vi "Configure FP-Message-Image.vi"(5 "header ref":refnum<vi>, 7 "Pop Up ref":refnum<vi>, 8 "error in (no error)":errorcluster, 9 "Image ref":refnum<vi>, 10 "Message ref":refnum<vi>, 11 "Popup in":refnum<class "Popup.lvclass">) -> (0 "error out":errorcluster, 2 "Panel Ref":refnum<vi>, 3 "Popup out":refnum<class "Popup.lvclass">, 4 "Panel Width":i32, 6 "Panel Height":i32)   [LabVIEW 2021, in "Pop-Up.lvlib" / "Popup.lvclass"]
doc: "Configure the front panel size, the message, and the image for a custom pop up type.\n\n<b>Code Developed By:</b>\nTechnology Service Corporation\n1983 S Liberty Drive\nBloomington, IN 47403\nPhone: 812 558-7100\nwww.tsc.com/atcs\n\nDeveloper:\nDaniel Coons"
uses:
  Popup.lvclass
  Popup.lvclass/Popup.ctl
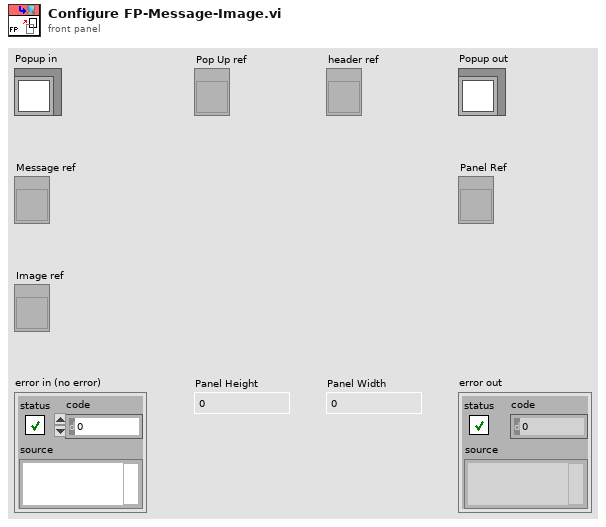
[diagram p1: front panel]
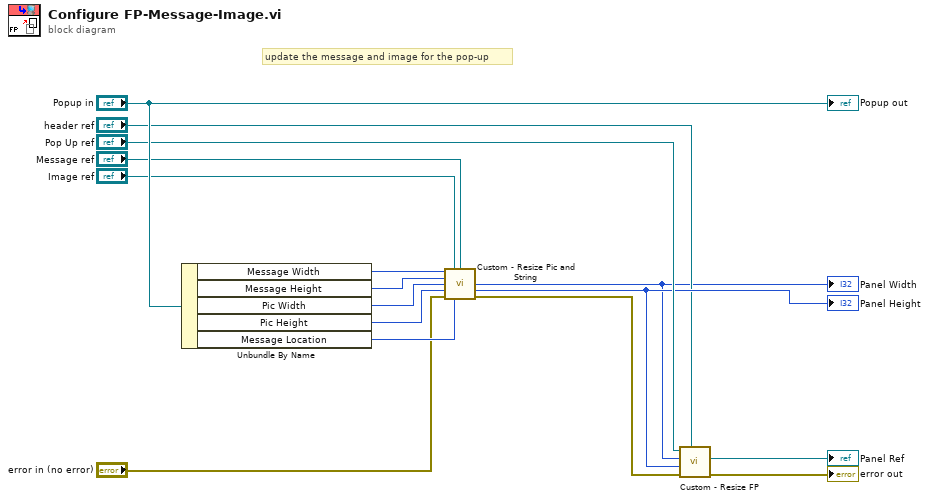
[diagram p0: block diagram]
diagram:
  # "update the message and image for the pop-up"
  n1 = Unbundle By Name("Popup in") -> ("Message Width"=w11:i32, "Message Height"=w12:i32, "Pic Width"=w13:i16, "Pic Height"=w14:i16, "Message Location"=w10:enum16{"Top", "Bottom", "Right", "Left"})
  n2 = call "Custom - Resize Pic and String.vi"("m.width"=w11, "2D Picture"="Image ref", "message ref"="Message ref", "m.height"=w12, "p.width"=w13, "p.height"=w14, "error in (no error)"="error in (no error)", "Message Location"=w10) -> ("Panel Width"=w1:i32, "Panel Height"=w5:i32, "error out"=w2:errorcluster)  [unwired: 5 in]
  "Panel Height" <- w5
  "Panel Width" <- w1
  n3 = call "Custom - Resize FP.vi"("header ref"="header ref", "error in (no error)"=w2, "Panel Height"=w5, "Panel Width"=w1, "VI in"="Pop Up ref") -> ("error out"=→"error out":errorcluster, "Panel Ref"=→"Panel Ref":refnum<vi>)  [unwired: 4 in, 1 out]
  "Popup out" <- "Popup in"
